vi "PASS_FAIL_Prompt.vi"(11 "Result":bool=TRUE) -> ()   [LabVIEW 2021]
uses:
  <vilib>/Utility/miscctls.llb/LVKeyNavTypeDef.ctl
panel:
  in  "String":string="press RED BUTTON on Jig to Unlock"
  in  "Pass":bool
  in  "Fail":bool
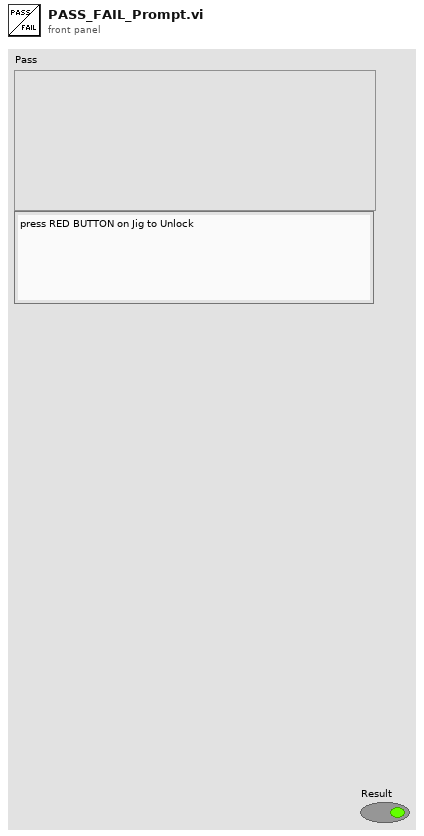
[diagram p1: front panel]
types:
  T1 = typedef "LVKeyNavTypeDef.ctl" = cluster{"Control":bool, "Shift":bool, "Key":string}
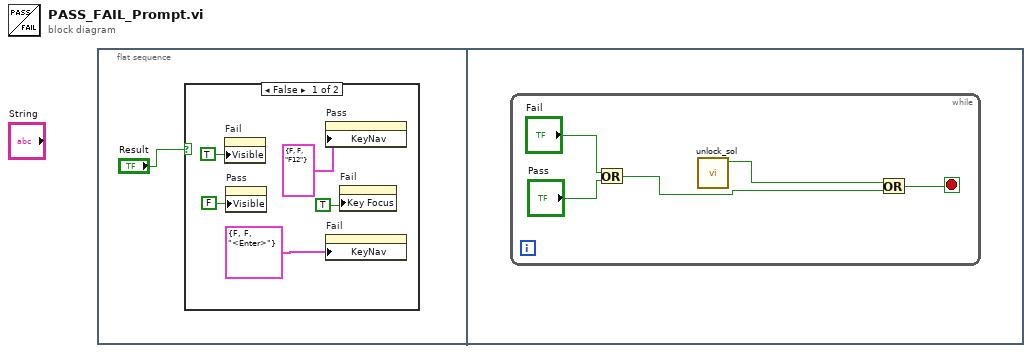
[diagram p0: block diagram]
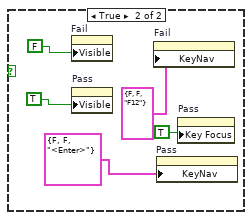
[diagram p2: hidden frame]
diagram:
  n1 = flat-sequence {
    frame #0 {
      n2 = case shown="False" "Result" {
        frame False {
          n3 = property on="Fail" class="Bool"("Visible"=TRUE) -> ()  [unwired: 2 in, 2 out]
          n4 = property on="Pass" class="Bool"("Visible"=FALSE) -> ()  [unwired: 2 in, 2 out]
          n5 = property on="Pass" class="Bool"("KeyNav"=T1 {"Control"=FALSE, "Shift"=FALSE, "Key"="F12"} ("Focus Key Binding")) -> ()  [unwired: 2 in, 2 out]
          n6 = property on="Fail" class="Bool"("KeyNav"=T1 {"Control"=FALSE, "Shift"=FALSE, "Key"="<Enter>"} ("Focus Key Binding")) -> ()  [unwired: 2 in, 2 out]
          n7 = property on="Fail" class="Bool"("Key Focus"=TRUE) -> ()  [unwired: 2 in, 2 out]
        }
        frame True {
          n8 = property on="Fail" class="Bool"("Visible"=FALSE) -> ()  [unwired: 2 in, 2 out]
          n9 = property on="Pass" class="Bool"("Visible"=TRUE) -> ()  [unwired: 2 in, 2 out]
          n10 = property on="Fail" class="Bool"("KeyNav"=T1 {"Control"=FALSE, "Shift"=FALSE, "Key"="F12"} ("Focus Key Binding")) -> ()  [unwired: 2 in, 2 out]
          n11 = property on="Pass" class="Bool"("KeyNav"=T1 {"Control"=FALSE, "Shift"=FALSE, "Key"="<Enter>"} ("Focus Key Binding")) -> ()  [unwired: 2 in, 2 out]
          n12 = property on="Pass" class="Bool"("Key Focus"=TRUE) -> ()  [unwired: 2 in, 2 out]
        }
      }
    }
    frame #1 {
      n13 = while {
        stop <- w14 stop-if-true
        n14 = Or(x="Fail", y="Pass") -> (x .or. y?=w12:bool)
        n15 = call "unlock_sol.vi"() -> ("Boolean"=w13:bool)  [unwired: 11 in]
        n16 = Or(x=w13, y=w12) -> (x .or. y?=w14:bool)
      }
    }
  }
